vi "ConvertToPosAnd3Currents.vi"(10 "dataFrame":u8[](array[numeric])) -> (2 "DblArray":sgl[](array[numeric]))   [LabVIEW 2017]
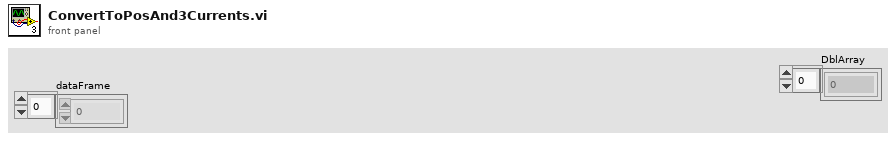
[diagram p1: front panel]
types:
  T1 = enum16{"big-endian, network order", "native, host order", "little-endian"}
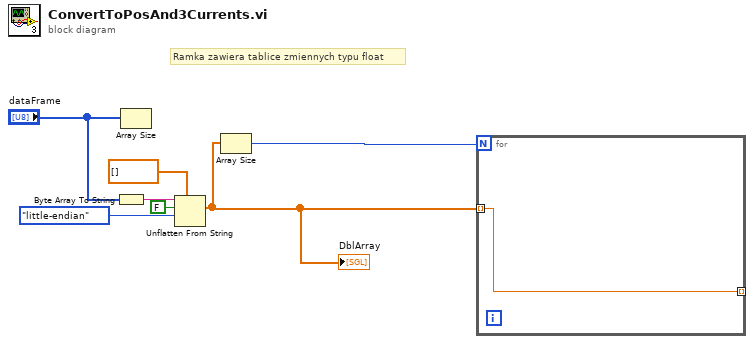
[diagram p0: block diagram]
diagram:
  # "Ramka zawiera tablice zmiennych typu float"
  n1 = Byte Array To String(unsigned byte array="dataFrame") -> (string=w7:string)
  n2 = Array Size(array="dataFrame") -> ()  [unwired: 1 out]
  n3 = Unflatten From String(type=sgl[] [], binary string=w7, data includes array or string size? (T)=FALSE, byte order (0:big-endian, network order)=T1."little-endian") -> (value=w1:sgl[])  [unwired: 1 in, 2 out]
  "DblArray" <- w1
  n4 = Array Size(array=w1) -> (size(s)=w2:i32)
  n5 = for {
    N: w2 -> [_]
    tunnel: w1 -> [w8] mode=indexing
    tunnel: [w8] -> _ mode=indexing
  }
